vi "op_rel_v5.vi"() -> ()   [LabVIEW 2010]
panel:
  out "L9":bool
  out "L8":bool
  in  "Slide":u8(slide)=4 scale=0.0..9.0
  out "L0":bool=TRUE
  out "L1":bool=TRUE
  out "L2":bool=TRUE
  out "L3":bool=TRUE
  out "L4":bool=TRUE
  out "L5":bool
  out "L6":bool
  out "L7":bool
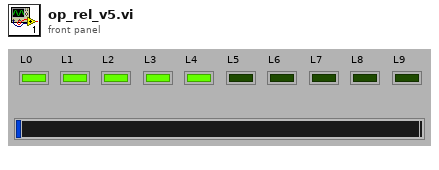
[diagram p1: front panel]
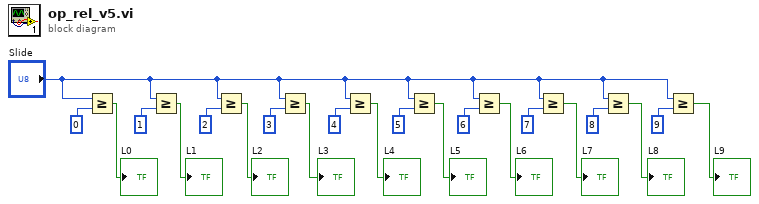
[diagram p0: block diagram]
diagram:
  n1 = Greater Or Equal?(x="Slide", y=0) -> (x >= y?=→"L0":bool)
  n2 = Greater Or Equal?(x="Slide", y=1) -> (x >= y?=→"L1":bool)
  n3 = Greater Or Equal?(x="Slide", y=2) -> (x >= y?=→"L2":bool)
  n4 = Greater Or Equal?(x="Slide", y=3) -> (x >= y?=→"L3":bool)
  n5 = Greater Or Equal?(x="Slide", y=4) -> (x >= y?=→"L4":bool)
  n6 = Greater Or Equal?(x="Slide", y=5) -> (x >= y?=→"L5":bool)
  n7 = Greater Or Equal?(x="Slide", y=6) -> (x >= y?=→"L6":bool)
  n8 = Greater Or Equal?(x="Slide", y=7) -> (x >= y?=→"L7":bool)
  n9 = Greater Or Equal?(x="Slide", y=8) -> (x >= y?=→"L8":bool)
  n10 = Greater Or Equal?(x="Slide", y=9) -> (x >= y?=→"L9":bool)
